vi "CO2 Limit Check.vi"(10 "54-55 Minutes (CO2)":dbl[](array[numeric]), 11 "24-25 Minutes (CO2)":dbl[](array[numeric])) -> (3 "CO2 In Spec":bool)   [LabVIEW 2020]
uses:
  <vilib>/Analysis/baseanly.llb/Mean (DBL).vi
  <vilib>/Analysis/NI_AALBase.lvlib
panel:
  out "24-25 Minutes (Lower Limit)":dbl format="%0.2f"
  out "24-25 Minutes (Upper Limit)":dbl format="%0.2f"
  out "54-55 Minutes (CO2) - Avg":dbl format="%0.2f"
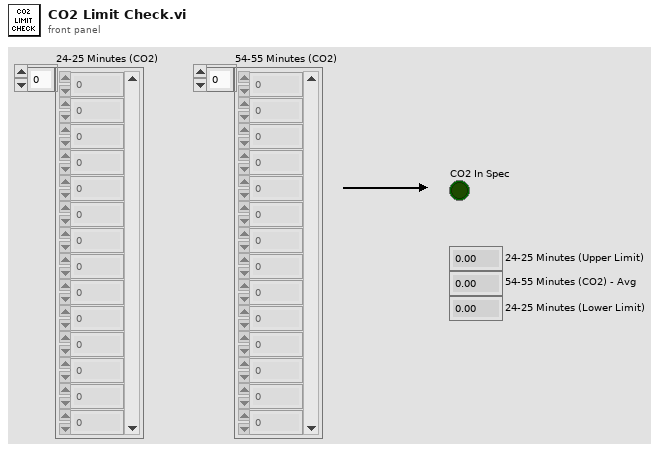
[diagram p1: front panel]
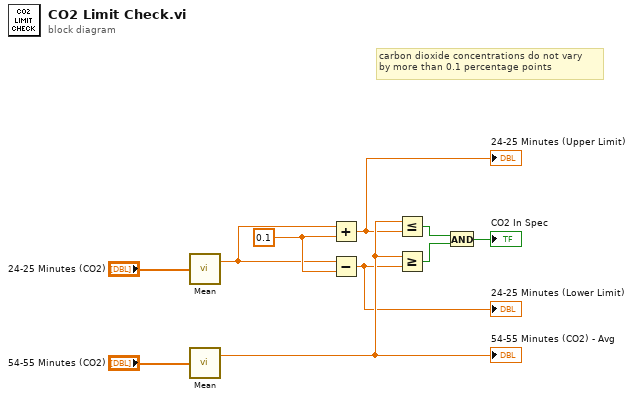
[diagram p0: block diagram]
diagram:
  w6 = 0.1 ("y")
  # "carbon dioxide concentrations do not vary\nby more than 0.1 percentage points"
  n1 = call-poly <vilib>:"Mean.vi"("X"="24-25 Minutes (CO2)") -> ("mean"=w5:dbl)  [unwired: 1 out]
  n2 = call-poly <vilib>:"Mean.vi"("X"="54-55 Minutes (CO2)") -> ("mean"=w10:dbl)  [unwired: 1 out]
  "54-55 Minutes (CO2) - Avg" <- w10
  n3 = Add(x=w5, y=w6) -> (x+y=w1:dbl)
  "24-25 Minutes (Upper Limit)" <- w1
  n4 = Subtract(x=w5, y=w6) -> (x-y=w2:dbl)
  "24-25 Minutes (Lower Limit)" <- w2
  n5 = Less Or Equal?(x=w10, y=w1) -> (x <= y?=w7:bool)
  n6 = Greater Or Equal?(x=w10, y=w2) -> (x >= y?=w8:bool)
  n7 = And(x=w7, y=w8) -> (x .and. y?=→"CO2 In Spec":bool)
